vi "Speed of Sound Freshwater.vi"(8 "Error In":errorcluster, 9 "Temperatures [C]":dbl[](array[numeric])) -> (0 "Error Out":errorcluster, 1 "Speed of Sound [m/s]":dbl[](array[numeric]) format="%_6g", 2 "Sensitivity [m/s/C]":dbl[](array[numeric]))   [LabVIEW 2016]
uses:
  <vilib>/Analysis/polynomials.llb/1D Polynomial Evaluation (DBL).vi
  <vilib>/Analysis/NI_AALPro.lvlib
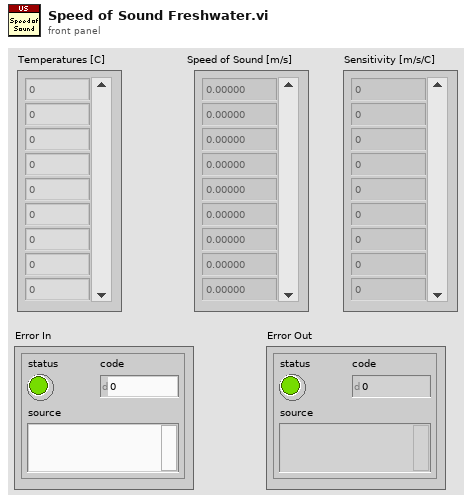
[diagram p1: front panel]
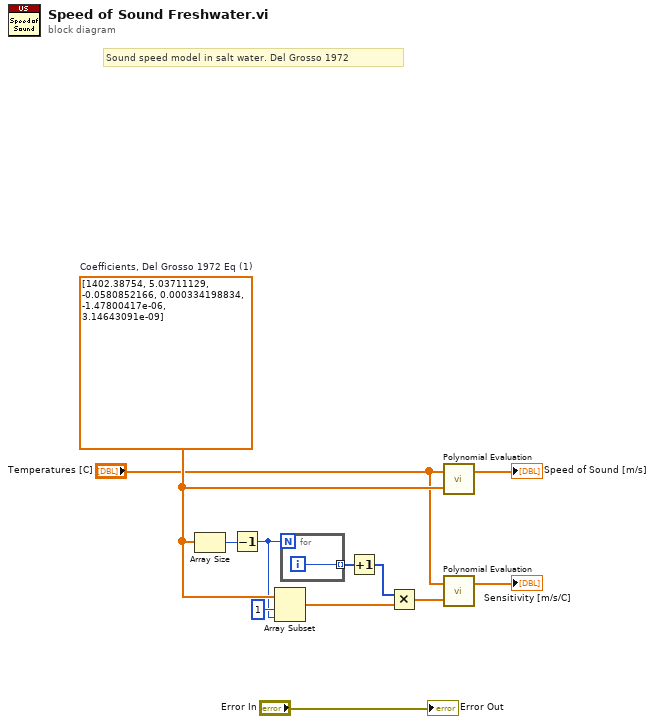
[diagram p0: block diagram]
diagram:
  w10 = dbl[] [1402.38754, 5.03711129, -0.0580852166, 0.000334198834, -1.47800417e-06, 3.14643091e-09]  # Coefficients, Del Grosso 1972 Eq (1)
  # "Sound speed model in salt water. Del Grosso 1972"
  n1 = Array Size(array=w10) -> (size(s)=w8:i32)
  n2 = Decrement(x=w8) -> (x-1=w7:i32)
  n3 = Array Subset(array=w10, index=1, length=w7) -> (w5:dbl[])
  n4 = for {
    N: w7 -> [_]
    tunnel: [w13] -> w6 mode=indexing
    i -> [w13]
  }
  n5 = Increment(x=w6) -> (x+1=w2:i32[])
  n6 = Multiply(x=w2, y=w5) -> (x*y=w3:dbl[])
  n7 = call-poly <vilib>:"Polynomial Evaluation.vi"("P(x)"=w10, "A"="Temperatures [C]") -> ("P(A)"=→"Speed of Sound [m/s]":dbl[])  [unwired: 1 out]
  n8 = call-poly <vilib>:"Polynomial Evaluation.vi"("P(x)"=w3, "A"="Temperatures [C]") -> ("P(A)"=→"Sensitivity [m/s/C]":dbl[])  [unwired: 1 out]
  "Error Out" <- "Error In"
